vi "Select Mode.vi"(0 "Mono1 Cut Enum":T7, 2 "Activation Type":T5(ring), 5 "Mono1 Coag Enum":T4, 7 "Mono2 Cut Enum":T3, 9 "Mono2 Coag Enum":T2, 11 "Bipolar Enum":T1) -> (4 "Change Mode Cluster":T6)   [LabVIEW 2024]
uses:
  Controls/Clusters/Change Mode Cluster.ctl
  Controls/Mode Enums/Mono1 Cut Enum.ctl
  Controls/Mode Enums/Mono1 Coag Enum.ctl
  Controls/Mode Enums/Mono2 Cut Enum.ctl
  Controls/Mode Enums/Mono2 Coag Enum.ctl
  Controls/Mode Enums/Bipolar Enum.ctl
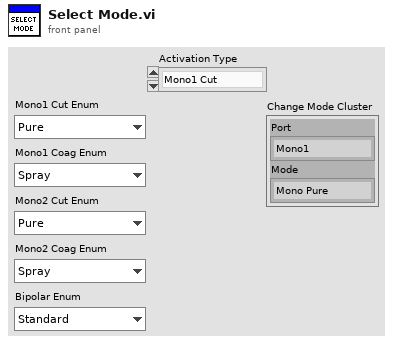
[diagram p1: front panel]
types:
  T1 = typedef "Bipolar Enum.ctl" = enum16{"Standard", "Macro", "Precision"}
  T2 = typedef "Mono2 Coag Enum.ctl" = enum16{"Spray", "Fulgerate"}
  T3 = typedef "Mono2 Cut Enum.ctl" = enum16{"Pure", "Blend"}
  T4 = typedef "Mono1 Coag Enum.ctl" = enum16{"Spray", "Fulgerate"}
  T5 = enum16{"Mono1 Cut", "Mono1 Coag", "Mono2 Cut", "Mono2 Coag", "Bipolar"}
  T6 = typedef "Change Mode Cluster.ctl" = cluster{"Port":enum16{"Mono1", "Mono2", "Bipolar", "Ligasure"}, "Mode":enum16{"Mono Pure", "Mono Blend", "Mono Fulgerate", "Mono Spray", "Bi Precision", "Bi Macro", "Bi Standard"}}
  T7 = typedef "Mono1 Cut Enum.ctl" = enum16{"Pure", "Blend"}
  T8 = enum16{"Mono Pure", "Mono Blend", "Mono Fulgerate", "Mono Spray", "Bi Precision", "Bi Macro", "Bi Standard"}
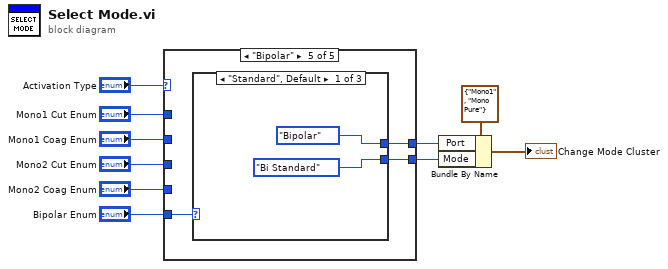
[diagram p0: block diagram]
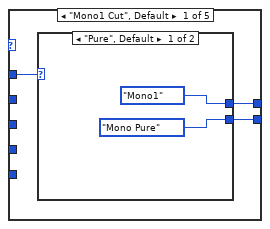
[diagram p2: hidden frame]
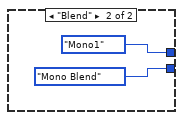
[diagram p3: hidden frame]
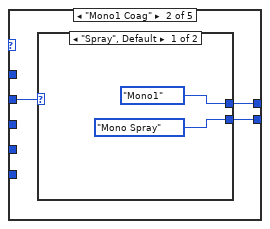
[diagram p4: hidden frame]
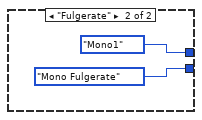
[diagram p5: hidden frame]
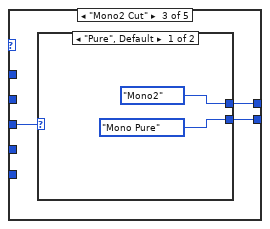
[diagram p6: hidden frame]
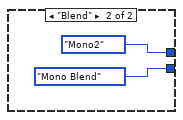
[diagram p7: hidden frame]
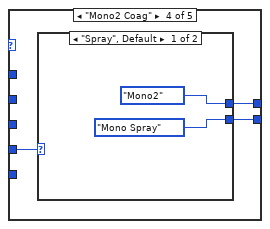
[diagram p8: hidden frame]
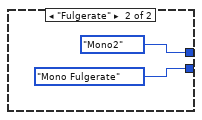
[diagram p9: hidden frame]
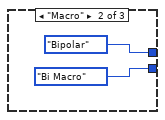
[diagram p10: hidden frame]
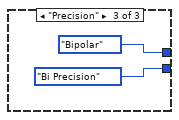
[diagram p11: hidden frame]
diagram:
  n1 = case shown="\"Bipolar\"" "Activation Type" {
    tunnel: [w12 w20 w27 w34 w41] -> w6
    tunnel: [w11 w19 w26 w33 w40] -> w5
    tunnel: "Mono1 Cut Enum" -> [w13 _ _ _ _]
    tunnel: "Mono1 Coag Enum" -> [_ w18 _ _ _]
    tunnel: "Mono2 Cut Enum" -> [_ _ w25 _ _]
    tunnel: "Mono2 Coag Enum" -> [_ _ _ w32 _]
    tunnel: "Bipolar Enum" -> [_ _ _ _ w39]
    frame "Mono1 Cut", Default {
      n2 = case shown="\"Pure\", Default" w13 {
        tunnel: [enum16{"Mono1", "Mono2", "Bipolar", "Ligasure"}."Mono1" ("Port") enum16{"Mono1", "Mono2", "Bipolar", "Ligasure"}."Mono1" ("Port")] -> w12
        tunnel: [T8."Mono Pure" ("Mode") T8."Mono Blend" ("Mode")] -> w11
        frame "Pure", Default {
        }
        frame "Blend" {
        }
      }
    }
    frame "Mono1 Coag" {
      n3 = case shown="\"Spray\", Default" w18 {
        tunnel: [enum16{"Mono1", "Mono2", "Bipolar", "Ligasure"}."Mono1" ("Port") enum16{"Mono1", "Mono2", "Bipolar", "Ligasure"}."Mono1" ("Port")] -> w20
        tunnel: [T8."Mono Spray" ("Mode") T8."Mono Fulgerate" ("Mode")] -> w19
        frame "Spray", Default {
        }
        frame "Fulgerate" {
        }
      }
    }
    frame "Mono2 Cut" {
      n4 = case shown="\"Pure\", Default" w25 {
        tunnel: [enum16{"Mono1", "Mono2", "Bipolar", "Ligasure"}."Mono2" ("Port") enum16{"Mono1", "Mono2", "Bipolar", "Ligasure"}."Mono2" ("Port")] -> w27
        tunnel: [T8."Mono Pure" ("Mode") T8."Mono Blend" ("Mode")] -> w26
        frame "Pure", Default {
        }
        frame "Blend" {
        }
      }
    }
    frame "Mono2 Coag" {
      n5 = case shown="\"Spray\", Default" w32 {
        tunnel: [enum16{"Mono1", "Mono2", "Bipolar", "Ligasure"}."Mono2" ("Port") enum16{"Mono1", "Mono2", "Bipolar", "Ligasure"}."Mono2" ("Port")] -> w34
        tunnel: [T8."Mono Spray" ("Mode") T8."Mono Fulgerate" ("Mode")] -> w33
        frame "Spray", Default {
        }
        frame "Fulgerate" {
        }
      }
    }
    frame "Bipolar" {
      n6 = case shown="\"Standard\", Default" w39 {
        tunnel: [enum16{"Mono1", "Mono2", "Bipolar", "Ligasure"}."Bipolar" ("Port") enum16{"Mono1", "Mono2", "Bipolar", "Ligasure"}."Bipolar" ("Port") enum16{"Mono1", "Mono2", "Bipolar", "Ligasure"}."Bipolar" ("Port")] -> w41
        tunnel: [T8."Bi Standard" ("Mode") T8."Bi Macro" ("Mode") T8."Bi Precision" ("Mode")] -> w40
        frame "Standard", Default {
        }
        frame "Macro" {
        }
        frame "Precision" {
        }
      }
    }
  }
  n7 = Bundle By Name(cluster=T6 {"Port"=enum."Mono1", "Mode"=enum."Mono Pure"}, "Port"=w6, "Mode"=w5) -> (→"Change Mode Cluster":T6)
